vi "Resume Panel Updates.vi"(8 "error in (no error)":errorcluster, 11 "PieChart in":refnum<class "PieChart.lvclass">) -> (0 "error out":errorcluster, 3 "PieChart out":refnum<class "PieChart.lvclass">)   [LabVIEW 2020, in "PieChart.lvclass"]
uses:
  PieChart.lvclass
  PieChart.lvclass/PieChart.ctl
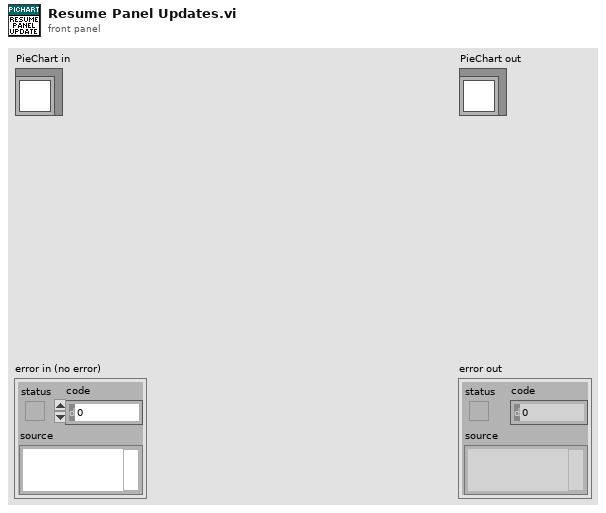
[diagram p1: front panel]
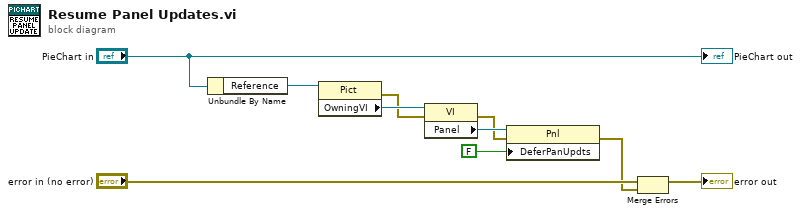
[diagram p0: block diagram]
diagram:
  n1 = Unbundle By Name("PieChart in") -> ("Reference"=w8:refnum<vi>)
  n2 = property class="Pict"(reference=w8) -> (error out=w6:errorcluster, "OwningVI"=w7:refnum<vi>)  [unwired: 1 in, 1 out]
  n3 = property class="VI"(reference=w7, error in=w6) -> (error out=w3:errorcluster, "Panel"=w5:refnum<vi>)  [unwired: 1 out]
  n4 = property class="Pnl"(reference=w5, error in=w3, "DeferPanUpdts"=FALSE ("Defer Panel Updates")) -> (error out=w1:errorcluster)  [unwired: 1 out]
  n5 = Merge Errors("error in (no error)", w1) -> (→"error out":errorcluster)
  "PieChart out" <- "PieChart in"
